vi "Optimization Tester.vi"(8 "error in":errorcluster, 11 "queue in":refnum<queue>) -> (0 "error out":errorcluster)   [LabVIEW 2018]
uses:
  Optimization/Generic Optimization Actor/Generic Optimization/Controls/Optimization Results Cluster.ctl
  Optimization/Generic Optimization Actor/Generic Optimization/Controls/Optimization Data Cluster.ctl
  Optimization/Generic Optimization Actor/Generic Optimization/Generic Optimization.lvclass
panel:
  in  "Optimization Data":T1
  out "return value":T2
  out "error out":errorcluster
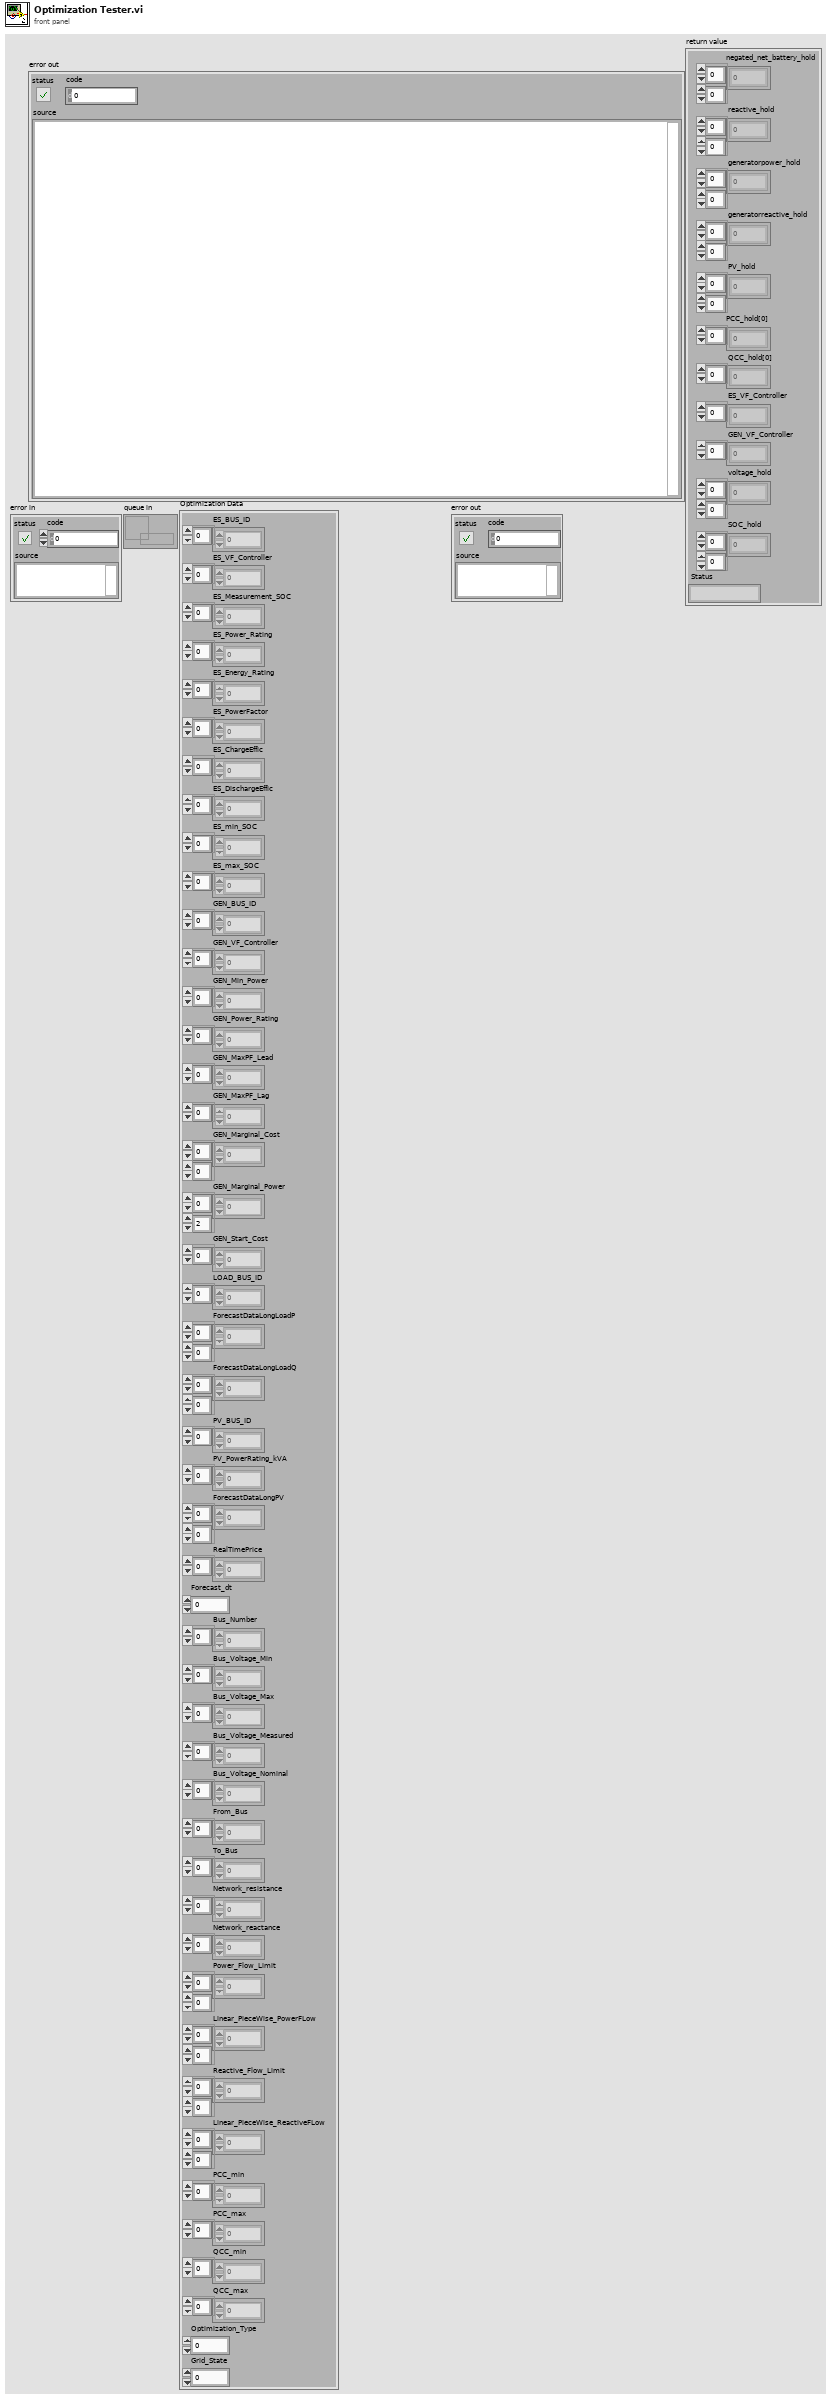
[diagram p1: front panel]
types:
  T1 = cluster{"ES_BUS_ID":dbl[], "ES_VF_Controller":dbl[], "ES_Measurement_SOC":dbl[], "ES_Power_Rating":dbl[], "ES_Energy_Rating":dbl[], "ES_PowerFactor":dbl[], "ES_ChargeEffic":dbl[], "ES_DischargeEffic":dbl[], "ES_min_SOC":dbl[], "ES_max_SOC":dbl[], "GEN_BUS_ID":dbl[], "GEN_VF_Controller":dbl[], "GEN_Min_Power":dbl[], "GEN_Power_Rating":dbl[], "GEN_MaxPF_Lead":dbl[], "GEN_MaxPF_Lag":dbl[], "GEN_Marginal_Cost":dbl[][], "GEN_Marginal_Power":dbl[][], "GEN_Start_Cost":dbl[], "LOAD_BUS_ID":dbl[], "ForecastDataLongLoadP":dbl[][], "ForecastDataLongLoadQ":dbl[][], "PV_BUS_ID":dbl[], "PV_PowerRating_kVA":dbl[], "ForecastDataLongPV":dbl[][], "RealTimePrice":dbl[], "Forecast_dt":dbl, "Bus_Number":dbl[], "Bus_Voltage_Min":dbl[], "Bus_Voltage_Max":dbl[], "Bus_Voltage_Measured":dbl[], "Bus_Voltage_Nominal":dbl[], "From_Bus":dbl[], "To_Bus":dbl[], "Network_resistance":dbl[], "Network_reactance":dbl[], "Power_Flow_Limit":dbl[][], "Linear_PieceWise_PowerFLow":dbl[][], "Reactive_Flow_Limit":dbl[][], "Linear_PieceWise_ReactiveFLow":dbl[][], "PCC_min":dbl[], "PCC_max":dbl[], "QCC_min":dbl[], "QCC_max":dbl[], "Optimization_Type":i32, "Grid_State":i32}
  T2 = typedef "Generic Optimization Actor.lvlib/Generic Optimization.lvclass/Optimization Results Cluster.ctl" = cluster{"negated_net_battery_hold":dbl[][], " reactive_hold":dbl[][], " generatorpower_hold":dbl[][], " generatorreactive_hold":dbl[][], " PV_hold":dbl[][], "PCC_hold[0]":dbl[], " QCC_hold[0]":dbl[], " ES_VF_Controller":dbl[], " GEN_VF_Controller":dbl[], " voltage_hold":dbl[][], " SOC_hold":dbl[][], " Status":string}
  T3 = typedef "Generic Optimization Actor.lvlib/Generic Optimization.lvclass/Optimization Data Cluster.ctl" = cluster{"ES_BUS_ID":dbl[], "ES_VF_Controller":dbl[], "ES_Measurement_SOC":dbl[], "ES_Power_Rating":dbl[], "ES_Energy_Rating":dbl[], "ES_PowerFactor":dbl[], "ES_ChargeEffic":dbl[], "ES_DischargeEffic":dbl[], "ES_min_SOC":dbl[], "ES_max_SOC":dbl[], "GEN_BUS_ID":dbl[], "GEN_VF_Controller":dbl[], "GEN_Min_Power":dbl[], "GEN_Power_Rating":dbl[], "GEN_MaxPF_Lead":dbl[], "GEN_MaxPF_Lag":dbl[], "GEN_Marginal_Cost":dbl[][], "GEN_Marginal_Power":dbl[][], "GEN_Start_Cost":dbl[], "LOAD_BUS_ID":dbl[], "ForecastDataLongLoadP":dbl[][], "ForecastDataLongLoadQ":dbl[][], "PV_BUS_ID":dbl[], "PV_PowerRating_kVA":dbl[], "ForecastDataLongPV":dbl[][], "RealTimePrice":dbl[], "Forecast_dt":dbl, "Bus_Number":dbl[], "Bus_Voltage_Min":dbl[], "Bus_Voltage_Max":dbl[], "Bus_Voltage_Measured":dbl[], "Bus_Voltage_Nominal":dbl[], "From_Bus":dbl[], "To_Bus":dbl[], "Network_resistance":dbl[], "Network_reactance":dbl[], "Power_Flow_Limit":dbl[][], "Linear_PieceWise_PowerFLow":dbl[][], "Reactive_Flow_Limit":dbl[][], "Linear_PieceWise_ReactiveFLow":dbl[][], "PCC_min":dbl[], "PCC_max":dbl[], "QCC_min":dbl[], "QCC_max":dbl[], "Optimization_Type":i32, "Grid_State":i32}
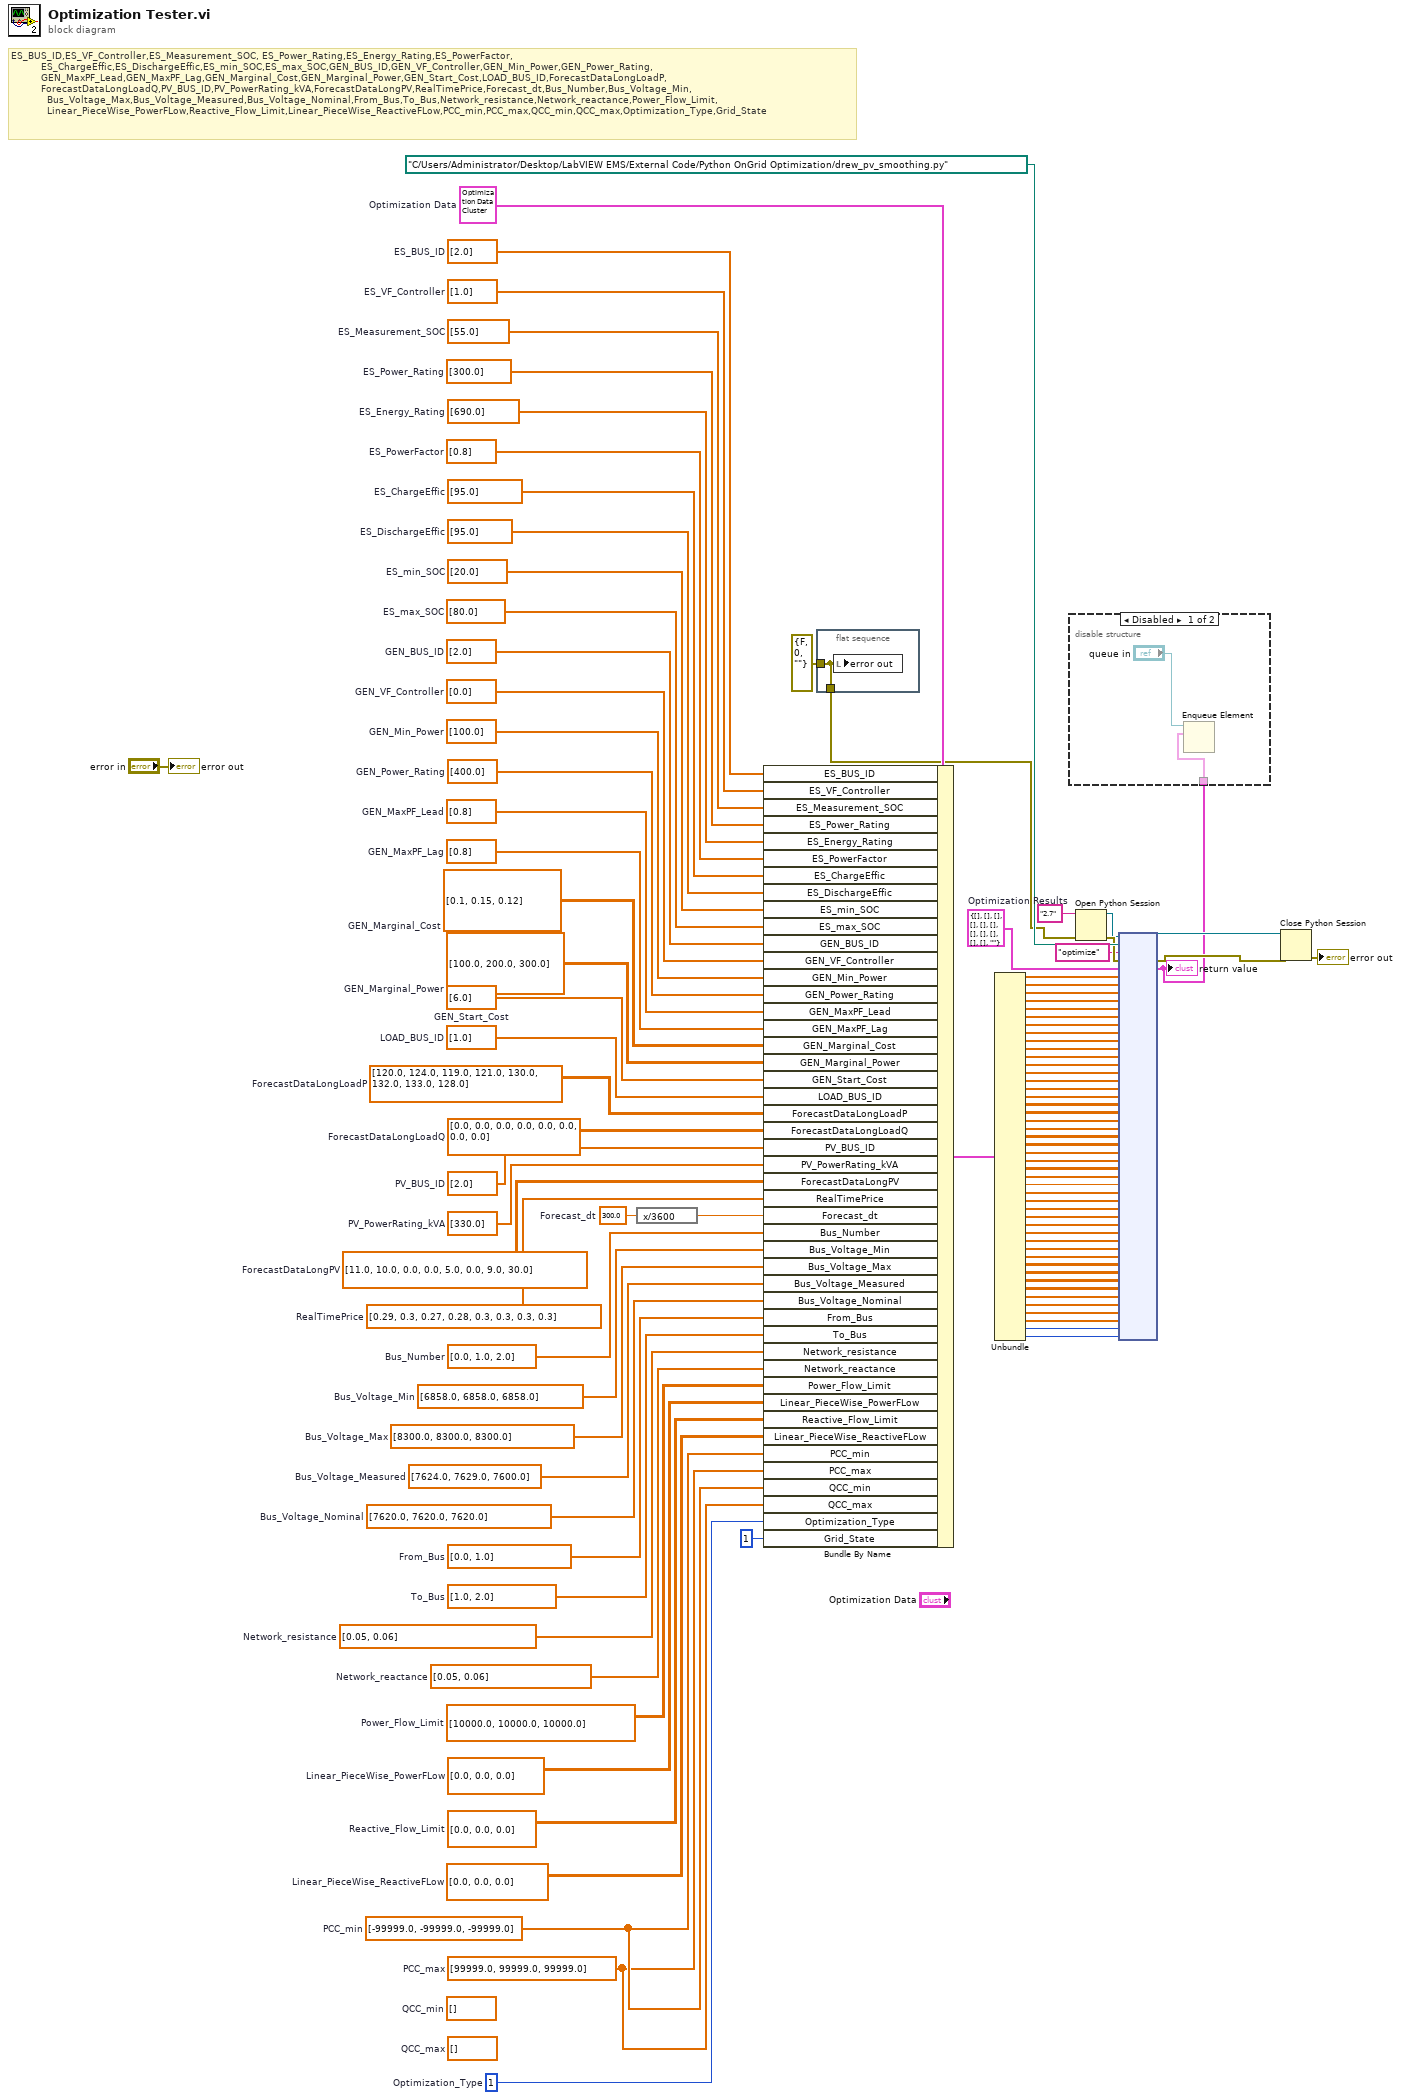
[diagram p0: block diagram]
diagram:
  w9 = T2 {"negated_net_battery_hold"=[], " reactive_hold"=[], " generatorpower_hold"=[], " generatorreactive_hold"=[], " PV_hold"=[], "PCC_hold[0]"=[], " QCC_hold[0]"=[], " ES_VF_Controller"=[], " GEN_VF_Controller"=[], " voltage_hold"=[], " SOC_hold"=[], " Status"=""}  # Optimization Results
  w64 = 1  # Optimization_Type
  (unwired) dbl[] []  # QCC_max
  (unwired) dbl[] []  # QCC_min
  w10 = dbl[] [99999.0, 99999.0, 99999.0]  # PCC_max
  w11 = dbl[] [-99999.0, -99999.0, -99999.0]  # PCC_min
  w65 = dbl[][] [[0.0, 0.0, 0.0]]  # Linear_PieceWise_ReactiveFLow
  w66 = dbl[][] [[0.0, 0.0, 0.0]]  # Reactive_Flow_Limit
  w67 = dbl[][] [[0.0, 0.0, 0.0]]  # Linear_PieceWise_PowerFLow
  w68 = dbl[][] [[10000.0, 10000.0, 10000.0]]  # Power_Flow_Limit
  w69 = dbl[] [0.05, 0.06]  # Network_reactance
  w70 = dbl[] [0.05, 0.06]  # Network_resistance
  w71 = dbl[] [1.0, 2.0]  # To_Bus
  w72 = dbl[] [0.0, 1.0]  # From_Bus
  w73 = dbl[] [7620.0, 7620.0, 7620.0]  # Bus_Voltage_Nominal
  w74 = dbl[] [7624.0, 7629.0, 7600.0]  # Bus_Voltage_Measured
  w75 = dbl[] [8300.0, 8300.0, 8300.0]  # Bus_Voltage_Max
  w76 = dbl[] [6858.0, 6858.0, 6858.0]  # Bus_Voltage_Min
  w77 = dbl[] [0.0, 1.0, 2.0]  # Bus_Number
  w3 = 300.0  # Forecast_dt
  w78 = dbl[] [0.29, 0.3, 0.27, 0.28, 0.3, 0.3, 0.3, 0.3]  # RealTimePrice
  w79 = dbl[][] [[11.0, 10.0, 0.0, 0.0, 5.0, 0.0, 9.0, 30.0]]  # ForecastDataLongPV
  w80 = dbl[] [330.0]  # PV_PowerRating_kVA
  w81 = dbl[] [2.0]  # PV_BUS_ID
  w82 = dbl[][] [[0.0, 0.0, 0.0, 0.0, 0.0, 0.0, 0.0, 0.0]]  # ForecastDataLongLoadQ
  w83 = dbl[][] [[120.0, 124.0, 119.0, 121.0, 130.0, 132.0, 133.0, 128.0]]  # ForecastDataLongLoadP
  w84 = dbl[] [1.0]  # LOAD_BUS_ID
  w85 = dbl[] [6.0]  # GEN_Start_Cost
  w86 = dbl[][] [[100.0, 200.0, 300.0]]  # GEN_Marginal_Power
  w87 = dbl[][] [[0.1, 0.15, 0.12]]  # GEN_Marginal_Cost
  w88 = dbl[] [0.8]  # GEN_MaxPF_Lag
  w89 = dbl[] [0.8]  # GEN_MaxPF_Lead
  w90 = dbl[] [400.0]  # GEN_Power_Rating
  w91 = dbl[] [100.0]  # GEN_Min_Power
  w92 = dbl[] [0.0]  # GEN_VF_Controller
  w93 = dbl[] [2.0]  # GEN_BUS_ID
  w94 = dbl[] [80.0]  # ES_max_SOC
  w95 = dbl[] [20.0]  # ES_min_SOC
  w96 = dbl[] [95.0]  # ES_DischargeEffic
  w97 = dbl[] [95.0]  # ES_ChargeEffic
  w98 = dbl[] [0.8]  # ES_PowerFactor
  w99 = dbl[] [690.0]  # ES_Energy_Rating
  w100 = dbl[] [300.0]  # ES_Power_Rating
  w101 = dbl[] [55.0]  # ES_Measurement_SOC
  w102 = dbl[] [1.0]  # ES_VF_Controller
  w103 = dbl[] [2.0]  # ES_BUS_ID
  w104 = T3 {"ES_BUS_ID"=[], "ES_VF_Controller"=[], "ES_Measurement_SOC"=[], "ES_Power_Rating"=[], "ES_Energy_Rating"=[], "ES_PowerFactor"=[], "ES_ChargeEffic"=[], "ES_DischargeEffic"=[], "ES_min_SOC"=[], "ES_max_SOC"=[], "GEN_BUS_ID"=[], "GEN_VF_Controller"=[], "GEN_Min_Power"=[], "GEN_Power_Rating"=[], "GEN_MaxPF_Lead"=[], "GEN_MaxPF_Lag"=[], "GEN_Marginal_Cost"=[], "GEN_Marginal_Power"=[], "GEN_Start_Cost"=[], "LOAD_BUS_ID"=[], "ForecastDataLongLoadP"=[], "ForecastDataLongLoadQ"=[], "PV_BUS_ID"=[], "PV_PowerRating_kVA"=[], "ForecastDataLongPV"=[], "RealTimePrice"=[], "Forecast_dt"=0.0, "Bus_Number"=[], "Bus_Voltage_Min"=[], "Bus_Voltage_Max"=[], "Bus_Voltage_Measured"=[], "Bus_Voltage_Nominal"=[], "From_Bus"=[], "To_Bus"=[], "Network_resistance"=[], "Network_reactance"=[], "Power_Flow_Limit"=[], "Linear_PieceWise_PowerFLow"=[], "Reactive_Flow_Limit"=[], "Linear_PieceWise_ReactiveFLow"=[], "PCC_min"=[], "PCC_max"=[], "QCC_min"=[], "QCC_max"=[], "Optimization_Type"=0, "Grid_State"=0}  # Optimization Data
  # "ES_BUS_ID,ES_VF_Controller,ES_Measurement_SOC, ES_Power_Rating,ES_Energy_Rating,ES_PowerFactor,\n          ES_ChargeEffic,ES_DischargeEffic,ES_min_SOC,ES_max_SOC,GEN_BUS_ID,GEN_VF_Controller,GEN_Min_Power,GEN_Power_Rating,\n          GEN_MaxPF_Lead,GEN_MaxPF_Lag,GEN_Marginal_Cost,GEN_Marginal_Power,GEN_Start_Cost,LOAD_BUS_ID,ForecastDataLongLoadP,\n          ForecastDataLongLoadQ,PV_BUS_ID,PV_PowerRating_kVA,ForecastDataLongPV,RealTimePrice,Forecast_dt,Bus_Number,Bus_Voltage_Min,\n            Bus_Voltage_Max,Bus_Voltage_Measured,Bus_Voltage_Nominal,From_Bus,To_Bus,Network_resistance,Network_reactance,Power_Flow_Limit,\n            Linear_PieceWise_PowerFLow,Reactive_Flow_Limit,Linear_PieceWise_ReactiveFLow,PCC_min,PCC_max,QCC_min,QCC_max,Optimization_Type,Grid_State"
  n1 = expression code="x/3600"(w3) -> (w1:dbl)
  n2 = Bundle By Name(cluster=w104, "ES_BUS_ID"=w103, "ES_VF_Controller"=w102, "ES_Measurement_SOC"=w101, "ES_Power_Rating"=w100, "ES_Energy_Rating"=w99, "ES_PowerFactor"=w98, "ES_ChargeEffic"=w97, "ES_DischargeEffic"=w96, "ES_min_SOC"=w95, "ES_max_SOC"=w94, "GEN_BUS_ID"=w93, "GEN_VF_Controller"=w92, "GEN_Min_Power"=w91, "GEN_Power_Rating"=w90, "GEN_MaxPF_Lead"=w89, "GEN_MaxPF_Lag"=w88, "GEN_Marginal_Cost"=w87, "GEN_Marginal_Power"=w86, "GEN_Start_Cost"=w85, "LOAD_BUS_ID"=w84, "ForecastDataLongLoadP"=w83, "ForecastDataLongLoadQ"=w82, "PV_BUS_ID"=w81, "PV_PowerRating_kVA"=w80, "ForecastDataLongPV"=w79, "RealTimePrice"=w78, "Forecast_dt"=w1, "Bus_Number"=w77, "Bus_Voltage_Min"=w76, "Bus_Voltage_Max"=w75, "Bus_Voltage_Measured"=w74, "Bus_Voltage_Nominal"=w73, "From_Bus"=w72, "To_Bus"=w71, "Network_resistance"=w70, "Network_reactance"=w69, "Power_Flow_Limit"=w68, "Linear_PieceWise_PowerFLow"=w67, "Reactive_Flow_Limit"=w66, "Linear_PieceWise_ReactiveFLow"=w65, "PCC_min"=w11, "PCC_max"=w10, "QCC_min"=w11, "QCC_max"=w10, "Optimization_Type"=w64, "Grid_State"=1) -> (w4:T3)
  n3 = flat-sequence {
    tunnel: errorcluster {"status"=FALSE, "code"=0, "source"=""} ("error in (no error)") -> [w107]
    tunnel: [w107] -> w2
    frame #0 {
      n4 = local write "error out"(w107) -> ()
    }
  }
  n5 = Unbundle(w4) -> ("ES_BUS_ID"=w62:dbl[], "ES_VF_Controller"=w61:dbl[], "ES_Measurement_SOC"=w60:dbl[], "ES_Power_Rating"=w59:dbl[], "ES_Energy_Rating"=w58:dbl[], "ES_PowerFactor"=w57:dbl[], "ES_ChargeEffic"=w56:dbl[], "ES_DischargeEffic"=w55:dbl[], "ES_min_SOC"=w54:dbl[], "ES_max_SOC"=w53:dbl[], "GEN_BUS_ID"=w52:dbl[], "GEN_VF_Controller"=w51:dbl[], "GEN_Min_Power"=w50:dbl[], "GEN_Power_Rating"=w49:dbl[], "GEN_MaxPF_Lead"=w48:dbl[], "GEN_MaxPF_Lag"=w47:dbl[], "GEN_Marginal_Cost"=w46:dbl[][], "GEN_Marginal_Power"=w45:dbl[][], "GEN_Start_Cost"=w44:dbl[], "LOAD_BUS_ID"=w43:dbl[], "ForecastDataLongLoadP"=w42:dbl[][], "ForecastDataLongLoadQ"=w41:dbl[][], "PV_BUS_ID"=w40:dbl[], "PV_PowerRating_kVA"=w39:dbl[], "ForecastDataLongPV"=w38:dbl[][], "RealTimePrice"=w37:dbl[], "Forecast_dt"=w36:dbl, "Bus_Number"=w35:dbl[], "Bus_Voltage_Min"=w34:dbl[], "Bus_Voltage_Max"=w33:dbl[], "Bus_Voltage_Measured"=w32:dbl[], "Bus_Voltage_Nominal"=w30:dbl[], "From_Bus"=w31:dbl[], "To_Bus"=w29:dbl[], "Network_resistance"=w28:dbl[], "Network_reactance"=w27:dbl[], "Power_Flow_Limit"=w26:dbl[][], "Linear_PieceWise_PowerFLow"=w25:dbl[][], "Reactive_Flow_Limit"=w24:dbl[][], "Linear_PieceWise_ReactiveFLow"=w23:dbl[][], "PCC_min"=w22:dbl[], "PCC_max"=w21:dbl[], "QCC_min"=w20:dbl[], "QCC_max"=w19:dbl[], "Optimization_Type"=w18:i32, "Grid_State"=w17:i32)
  n6 = Open Python Session(python version="2.7" ("Python version"), 3:w2) -> (session out=w8:refnum<k35>, error out=w15:errorcluster)  [unwired: 1 in]
  n7 = node(w8, path "C:/Users/Administrator/Desktop/LabVIEW EMS/External Code/Python OnGrid Optimization/drew_pv_smoothing.py" ("module path"), "optimize" ("function name"), w15, w9, w62, w61, w60, w59, w58, w57, w56, w55, w54, w53, w52, w51, w50, w49, w48, w47, w46, w45, w44, w43, w42, w41, w40, w39, w38, w37, w36, w35, w34, w33, w32, w30, w31, w29, w28, w27, w26, w25, w24, w23, w22, w21, w20, w19, w18, w17) -> (w16:refnum<k35>, w14:errorcluster, w6:T2)  [unwired: 46 in, 2 out]
  "return value" <- w6
  n8 = disable-structure shown="Disabled" {
    disable-tunnel: w6 -> [w108 _]
    frame Disabled {
      n9 = Enqueue Element(queue="queue in", element=w108) -> ()  [unwired: 2 in, 3 out]
    }
    frame Enabled {
    }
  }
  n10 = Close Python Session(session in=w16, error in=w14) -> (11:→"error out":errorcluster)
  "error out" <- "error in"
